vi "newtest.vi"() -> ()   [LabVIEW 2016]
panel:
  in  "N":dbl=100000.0
  out "x-y":dbl=11.299950899992837
  out "initial time":dbl=99380.9332687
  in  "M":dbl=20.0
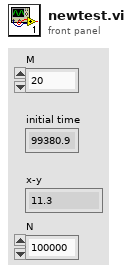
[diagram p1: front panel]
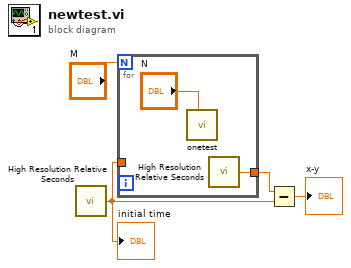
[diagram p0: block diagram]
diagram:
  n1 = call <vilib>:"High Resolution Relative Seconds.vi"() -> ("relative seconds"=w2:dbl)
  "initial time" <- w2
  n2 = for {
    N: "M" -> [_]
    tunnel: w2 -> [_]
    tunnel: [w6] -> w3
    n3 = call "onetest.vi"("N"="N") -> ()  [unwired: 11 in]
    n4 = call <vilib>:"High Resolution Relative Seconds.vi"() -> ("relative seconds"=w6:dbl)
  }
  n5 = Subtract(x=w3, y=w2) -> (x-y=→"x-y":dbl)
